vi "ParseArgumentsCore.vi"(8 "error in (no error)":errorcluster, 10 "Inputs":string[](array[string]), 11 "VIPMUninstallPackage in":refnum<class "VIPMUninstallPackage.lvclass">) -> (0 "error out":errorcluster, 3 "VIPMUninstallPackage out":refnum<class "VIPMUninstallPackage.lvclass">)   [LabVIEW 2014, in "VIPMUninstallPackage.lvclass"]
uses:
  <nishared>/LabVIEW CLI/Operations/VIPMUninstallPackage/VIPMUninstallPackage.lvclass
  <nishared>/LabVIEW CLI/Operations/Utilities/OperationErrorType.ctl
  <nishared>/LabVIEW CLI/Operations/VIPMUninstallPackage/VIPMUninstallPackage.lvclass/VIPMUninstallPackage.ctl
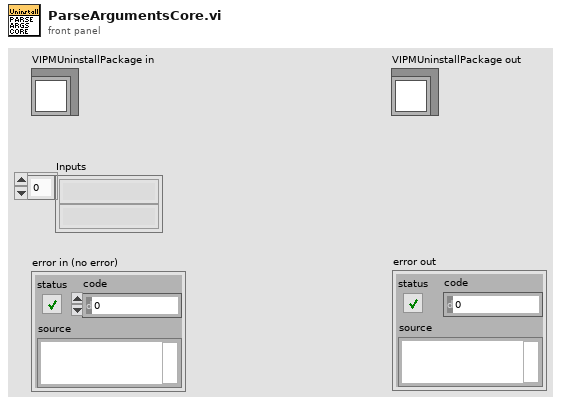
[diagram p1: front panel]
types:
  T1 = typedef "OperationErrorType.ctl" = enum16{"RequiredArgumentMissing", "UnknownArguments", "LoggerSetMultipleTimes", "OperationBrokenError"}
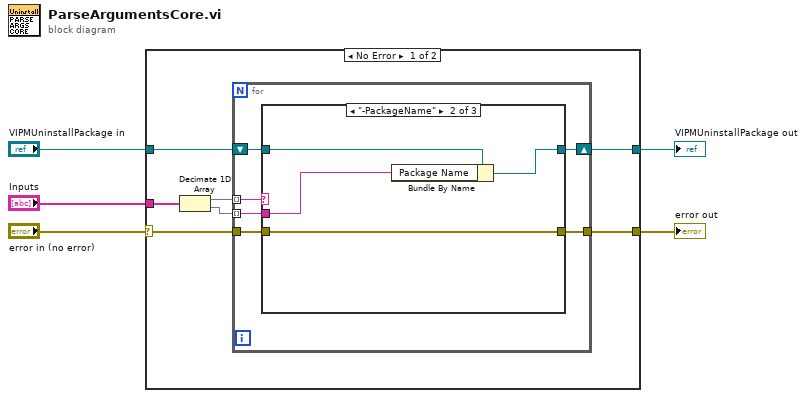
[diagram p0: block diagram]
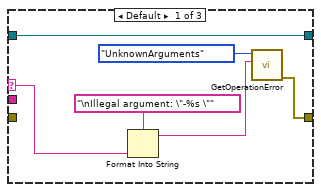
[diagram p2: hidden frame]
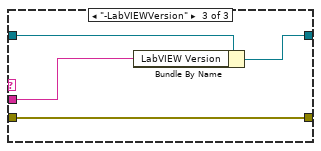
[diagram p3: hidden frame]
diagram:
  n1 = case shown="No Error" "error in (no error)" {
    selector: "error in (no error)" -> [w6 w34]
    tunnel: [w12 w34] -> w5
    tunnel: "Inputs" -> [w9 _]
    tunnel: "VIPMUninstallPackage in" -> [w8 w33]
    tunnel: [w7 w33] -> w2
    frame No Error {
      n2 = Decimate 1D Array(w9) -> (w10:string[], w11:string[])
      n3 = for {
        tunnel: w10 -> [w18] mode=indexing
        tunnel: w11 -> [w17] mode=indexing
        shift-right: [w15] -> w7
        shift-left: w8 -> [w16]
        tunnel: w6 -> [w14]
        tunnel: [w13] -> w12
        n4 = case shown="\"-PackageName\"" w18 {
          selector: w18 -> [w21 _ _]
          tunnel: w17 -> [_ w27 w31]
          tunnel: w16 -> [w24 w28 w32]
          tunnel: [w24 w26 w30] -> w15
          tunnel: w14 -> [_ w25 w29]
          tunnel: [w23 w25 w29] -> w13
          frame Default {
            n5 = Format Into String(format string="\nIllegal argument: \"-%s \"", w21) -> (resulting string=w19:string)  [unwired: 2 in, 1 out]
            n6 = call <nishared>:"GetOperationError.vi"("Additional Information"=w19, "Operation Error Type"=OperationErrorType."UnknownArguments") -> ("error out"=w23:errorcluster)  [unwired: 9 in]
          }
          frame "-PackageName" {
            n7 = Bundle By Name(cluster=w28, "Package Name"=w27) -> (w26:refnum<class "VIPMUninstallPackage.lvclass">)
          }
          frame "-LabVIEWVersion" {
            n8 = Bundle By Name(cluster=w32, "LabVIEW Version"=w31) -> (w30:refnum<class "VIPMUninstallPackage.lvclass">)
          }
        }
      }
    }
    frame Error {
    }
  }
  "error out" <- w5
  "VIPMUninstallPackage out" <- w2
